vi "Bank - Semaphore.vi"() -> ()   [LabVIEW 2012]
doc: "本VI模拟银行事务，演示竞争状态。\n\n运行本VI，尝试并发事务，观察存款或取款操作丢失的情况。尝试查找并解决该问题。"
panel:
  out "余额":dbl
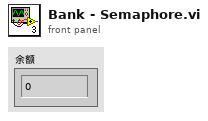
[diagram p1: front panel]
types:
  T1 = typedef "Account Info.ctl" = cluster{"银行集合点":T2, "取款队列":refnum<queue>, "存款队列":refnum<queue>}
  T2 = typedef "Rendezvous RefNum" = refnum<k1>
  T3 = typedef "Semaphore RefNum" = refnum<k1>
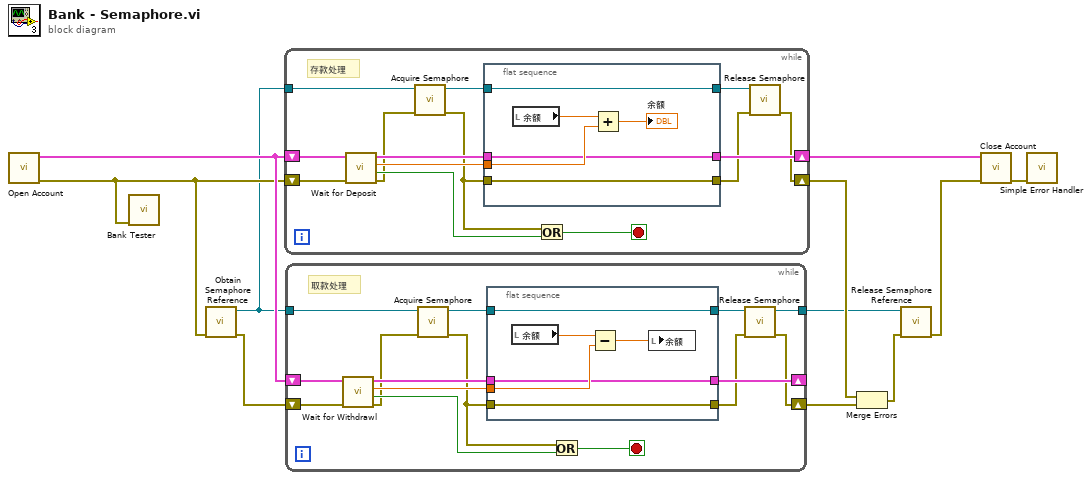
[diagram p0: block diagram]
diagram:
  n1 = call "Open Account.vi"() -> ("错误输出"=w6:errorcluster, "帐户信息"=w11:T1)  [unwired: 10 in]
  n2 = call "Bank Tester.vi"("错误输入"=w6) -> ()  [unwired: 10 in, 1 out]
  n3 = call <vilib>:"Obtain Semaphore Reference.vi"("error in (no error)"=w6) -> ("error out"=w5:errorcluster, "semaphore"=w1:T3)  [unwired: 4 in, 1 out]
  n4 = while {
    shift-right: [w21] -> w8
    shift-left: w11 -> [w24]
    shift-right: [w15] -> w10
    shift-left: w6 -> [w23]
    tunnel: w1 -> [w14]
    stop <- w19 stop-if-true
    # "存款处理"
    n5 = call "Wait for Deposit.vi"("错误输入"=w23, "帐户信息"=w24) -> ("错误输出"=w18:errorcluster, "停止？"=w20:bool, "存款额"=w25:dbl, "帐户信息输出"=w22:T1)  [unwired: 6 in]
    n6 = call <vilib>:"Acquire Semaphore.vi"("error in (no error)"=w18, "semaphore"=w14) -> ("error out"=w17:errorcluster, "semaphore out"=w13:T3)  [unwired: 3 in, 1 out]
    n7 = flat-sequence {
      tunnel: w25 -> [w31]
      tunnel: [w28] -> w21
      tunnel: w22 -> [w28]
      tunnel: w17 -> [w27]
      tunnel: [w27] -> w16
      tunnel: w13 -> [w26]
      tunnel: [w26] -> w12
      frame #0 {
        n8 = local read "余额"() -> (w29:dbl)
        n9 = Add ("加")(x=w29, y=w31) -> (x+y=→"余额":dbl)
      }
    }
    n10 = Or ("或")(x=w17, y=w20) -> (x .or. y?=w19:bool)
    n11 = call <vilib>:"Release Semaphore.vi"("error in (no error)"=w16, "semaphore"=w12) -> ("error out"=w15:errorcluster)  [unwired: 4 in, 1 out]
  }
  n12 = while {
    shift-right: [w42] -> _
    shift-left: w11 -> [w45]
    shift-right: [w32] -> w9
    shift-left: w5 -> [w44]
    tunnel: w1 -> [w39]
    tunnel: [w36] -> w2
    stop <- w40 stop-if-true
    # "取款处理"
    n13 = call "Wait for Withdrawl.vi"("错误输入"=w44, "帐户信息"=w45) -> ("错误输出"=w35:errorcluster, "停止？"=w41:bool, "取款额"=w46:dbl, "帐户信息输出"=w43:T1)  [unwired: 6 in]
    n14 = call <vilib>:"Acquire Semaphore.vi"("error in (no error)"=w35, "semaphore"=w39) -> ("error out"=w34:errorcluster, "semaphore out"=w38:T3)  [unwired: 3 in, 1 out]
    n15 = flat-sequence {
      tunnel: w46 -> [w50]
      tunnel: w43 -> [w49]
      tunnel: w34 -> [w48]
      tunnel: [w49] -> w42
      tunnel: [w48] -> w33
      tunnel: w38 -> [w47]
      tunnel: [w47] -> w37
      frame #0 {
        n16 = local read "余额"() -> (w51:dbl)
        n17 = Subtract ("减")(x=w51, y=w50) -> (x-y=w52:dbl)
        n18 = local write "余额"(w52) -> ()
      }
    }
    n19 = Or ("或")(x=w34, y=w41) -> (x .or. y?=w40:bool)
    n20 = call <vilib>:"Release Semaphore.vi"("error in (no error)"=w33, "semaphore"=w37) -> ("error out"=w32:errorcluster, "semaphore out"=w36:T3)  [unwired: 4 in]
  }
  n21 = Merge Errors ("合并错误")(w10, w9) -> (w4:errorcluster)
  n22 = call <vilib>:"Release Semaphore Reference.vi"("error in (no error)"=w4, "semaphore"=w2) -> ("error out"=w3:errorcluster)  [unwired: 8 in, 1 out]
  n23 = call "Close Account.vi"("错误输入"=w3, "帐户信息"=w8) -> ("错误输出"=w7:errorcluster)  [unwired: 9 in]
  n24 = call <vilib>:"Simple Error Handler.vi"("error in (no error)"=w7) -> ()  [unwired: 4 in, 5 out]
